vi "gun_lookup_speed.vi"(11 "Distance":dbl) -> (3 "Speed":dbl)   [LabVIEW 2011]
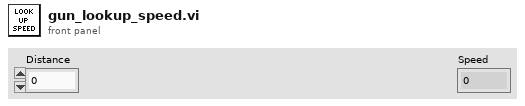
[diagram p1: front panel]
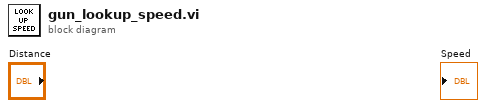
[diagram p0: block diagram]
diagram:
